vi "Manual Override.vi"(5 "Enable":bool, 7 "CMD Override":T1(ring)=enum."Shoot Speed", 8 "Velocity Data":dbl, 9 "Position Data":dbl, 10 "Percent Out Data":dbl, 11 "Auto CMD":T2) -> (3 "OverRide Command Out":T2)   [LabVIEW 2023, in "Shooter FX_ACT.lvlib"]
uses:
  Shooter FX_ACT.lvlib
  Cluster_CMD_ACT_Data.ctl
  ENUM_CMD_Mode Select.ctl
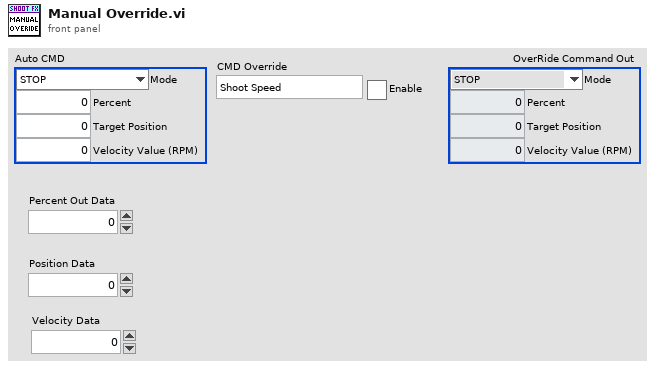
[diagram p1: front panel]
types:
  T1 = enum32{"Teleop-Auto", "Percent Output", "Position Value", "Velocity Value", "Shoot Speed", "STOP"}
  T2 = typedef "Shooter FX_ACT.lvlib/Cluster_CMD_ACT_Data.ctl" = cluster{"Mode":T3, "Percent":dbl, "Target Position":dbl, "Velocity Value (RPM)":dbl}
  T3 = typedef "Shooter FX_ACT.lvlib/ENUM_CMD_Mode Select.ctl" = enum16{"STOP", "PercentOut", "Positon Value", "Velocity Value", "Shoot Speed", "Auto Shoot"}
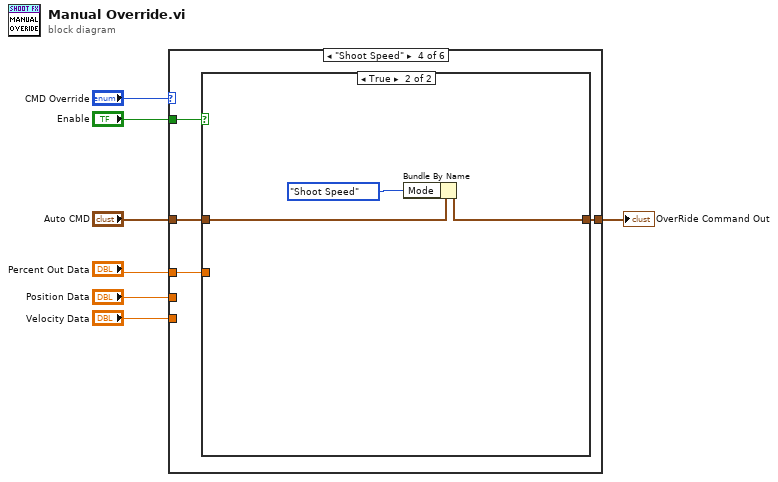
[diagram p0: block diagram]
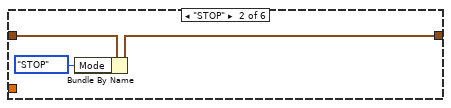
[diagram p3: hidden frame]
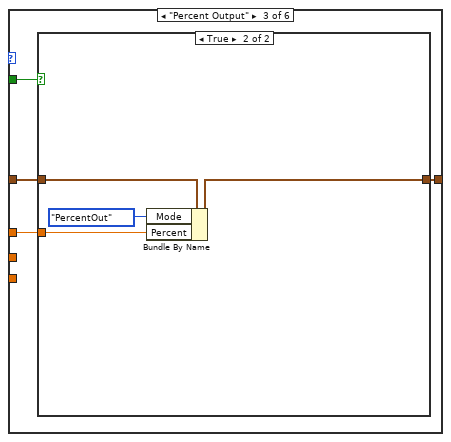
[diagram p4: hidden frame]
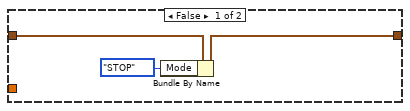
[diagram p5: hidden frame]
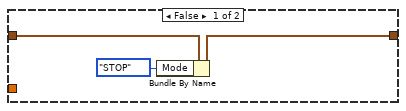
[diagram p6: hidden frame]
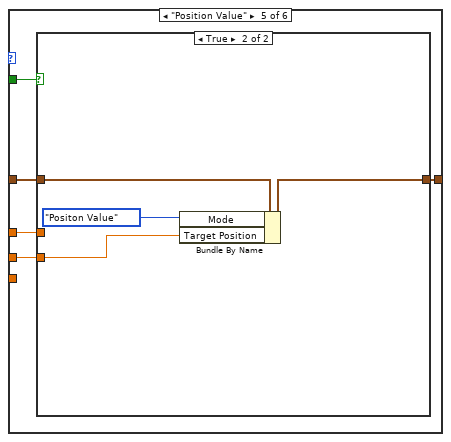
[diagram p7: hidden frame]
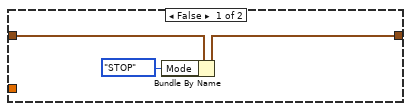
[diagram p8: hidden frame]
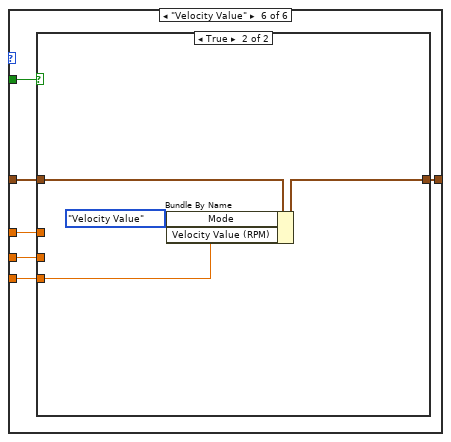
[diagram p9: hidden frame]
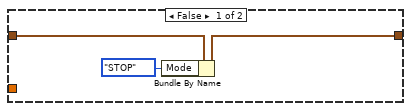
[diagram p10: hidden frame]
diagram:
  n1 = case shown="\"Shoot Speed\"" "CMD Override" {
    tunnel: [w8 w9 w14 w25 w36 w49] -> w7
    tunnel: "Auto CMD" -> [w8 w10 w15 w26 w37 w50]
    tunnel: "Enable" -> [_ _ w13 w24 w35 w48]
    tunnel: "Percent Out Data" -> [_ _ w12 w23 w34 w47]
    tunnel: "Position Data" -> [_ _ _ _ w33 w46]
    tunnel: "Velocity Data" -> [_ _ _ _ _ w45]
    frame "Teleop-Auto" {
    }
    frame "STOP" {
      n2 = Bundle By Name(cluster=w10, "Mode"=ENUM_CMD_Mode_Select."STOP") -> (w9:T2)
    }
    frame "Percent Output" {
      n3 = case shown="True" w13 {
        tunnel: w15 -> [w17 w22]
        tunnel: [w16 w20] -> w14
        tunnel: w12 -> [_ w19]
        frame False {
          n4 = Bundle By Name(cluster=w17, "Mode"=ENUM_CMD_Mode_Select."STOP") -> (w16:T2)
        }
        frame True {
          n5 = Bundle By Name(cluster=w22, "Mode"=ENUM_CMD_Mode_Select."PercentOut", "Percent"=w19) -> (w20:T2)
        }
      }
    }
    frame "Shoot Speed" {
      n6 = case shown="True" w24 {
        tunnel: w26 -> [w28 w32]
        tunnel: [w27 w30] -> w25
        tunnel: w23 -> [_ _]
        frame False {
          n7 = Bundle By Name(cluster=w28, "Mode"=ENUM_CMD_Mode_Select."STOP") -> (w27:T2)
        }
        frame True {
          n8 = Bundle By Name(cluster=w32, "Mode"=ENUM_CMD_Mode_Select."Shoot Speed") -> (w30:T2)
        }
      }
    }
    frame "Position Value" {
      n9 = case shown="True" w35 {
        tunnel: w37 -> [w39 w44]
        tunnel: [w38 w42] -> w36
        tunnel: w34 -> [_ _]
        tunnel: w33 -> [_ w41]
        frame False {
          n10 = Bundle By Name(cluster=w39, "Mode"=ENUM_CMD_Mode_Select."STOP") -> (w38:T2)
        }
        frame True {
          n11 = Bundle By Name(cluster=w44, "Mode"=ENUM_CMD_Mode_Select."Positon Value", "Target Position"=w41) -> (w42:T2)
        }
      }
    }
    frame "Velocity Value" {
      n12 = case shown="True" w48 {
        tunnel: w50 -> [w52 w57]
        tunnel: [w51 w55] -> w49
        tunnel: w47 -> [_ _]
        tunnel: w46 -> [_ _]
        tunnel: w45 -> [_ w54]
        frame False {
          n13 = Bundle By Name(cluster=w52, "Mode"=ENUM_CMD_Mode_Select."STOP") -> (w51:T2)
        }
        frame True {
          n14 = Bundle By Name(cluster=w57, "Mode"=ENUM_CMD_Mode_Select."Velocity Value", "Velocity Value (RPM)"=w54) -> (w55:T2)
        }
      }
    }
  }
  "OverRide Command Out" <- w7
